vi "UI Screen Updater.vi"(8 "error in (no error)":errorcluster, 11 "Range Updater Cntrl":T1) -> (0 "error out":errorcluster)   [LabVIEW 2018]
uses:
  Shared Controls/Range Updater.ctl
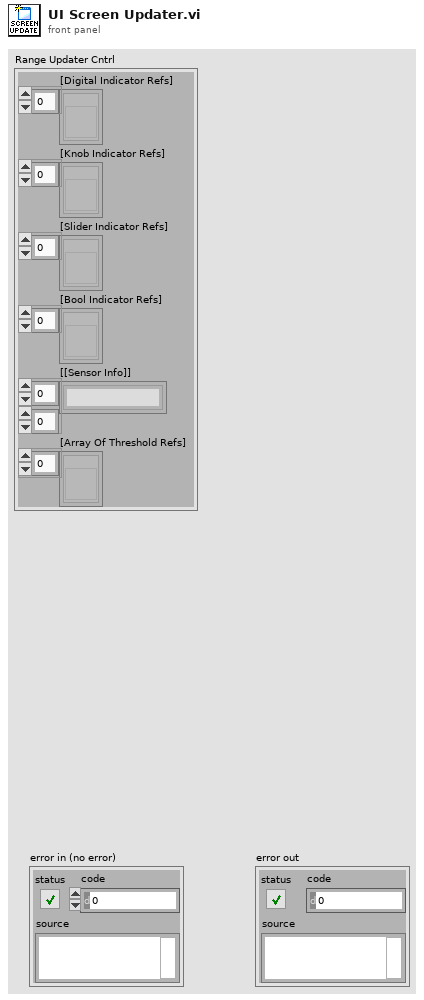
[diagram p1: front panel]
types:
  T1 = typedef "Range Updater.ctl" = cluster{"[Digital Indicator Refs]":refnum<vi>[], "[Knob Indicator Refs]":refnum<vi>[], "[Slider Indicator Refs]":refnum<vi>[], "[Bool Indicator Refs]":refnum<vi>[], "[[Sensor Info]]":string[][], "[Array Of Threshold Refs]":refnum<vi>[]}
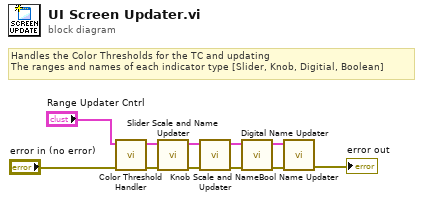
[diagram p0: block diagram]
diagram:
  # "Handles the Color Thresholds for the TC and updating\nThe ranges and names of each indicator type [Slider, Knob, Digitial, Boolean]"
  n1 = call "Color Threshold Handler.vi"("error in (no error)"="error in (no error)", "Range Updater Cntrl in"="Range Updater Cntrl") -> ("error out"=w6:errorcluster, "Range Updater Cntrl out"=w4:T1)  [unwired: 8 in]
  n2 = call "Slider Scale and Name Updater.vi"("error in (no error)"=w6, "Cluster In"=w4) -> ("error out"=w8:errorcluster, "Cluster Out"=w3:T1)  [unwired: 8 in]
  n3 = call "Knob Scale and Name Updater.vi"("error in"=w8, "Cluster In"=w3) -> ("error out"=w9:errorcluster, "Cluster out"=w2:T1)  [unwired: 8 in]
  n4 = call "Digital Name Updater.vi"("error in (no error)"=w9, "Cluster In"=w2) -> ("error out"=w10:errorcluster, "Cluster Out"=w1:T1)  [unwired: 8 in]
  n5 = call "Bool Name Updater.vi"("error in (no error)"=w10, "Cluster In"=w1) -> ("error out"=→"error out":errorcluster)  [unwired: 9 in]
